vi "Мажор.vi"() -> ()   [LabVIEW 2013]
panel:
  out "output array":dbl[](array[numeric])
  out "s? t:f":dbl
  out "element":dbl
  out "После ошибки":dbl[](array[numeric])
  out "2-х массив на выходе 3":dbl[][](array[numeric])
  out "x*y":i32
  out "size(s)":i32
  in  "Размер окна":i32=4
  out "см. 1.5":dbl[][](array[numeric])
  out "Декодированное сообщение":dbl[](array[numeric])
  out "Детектированное сообщение":dbl[](array[numeric])
  out "Numeric":dbl
  out "Numeric 2":dbl
  out "До ошибки":dbl[](array[numeric])
  in  "Кол-во копий":i32=5
  out "Массиве":dbl[](array[numeric])
  in  "Кол-во элементов":i32=16
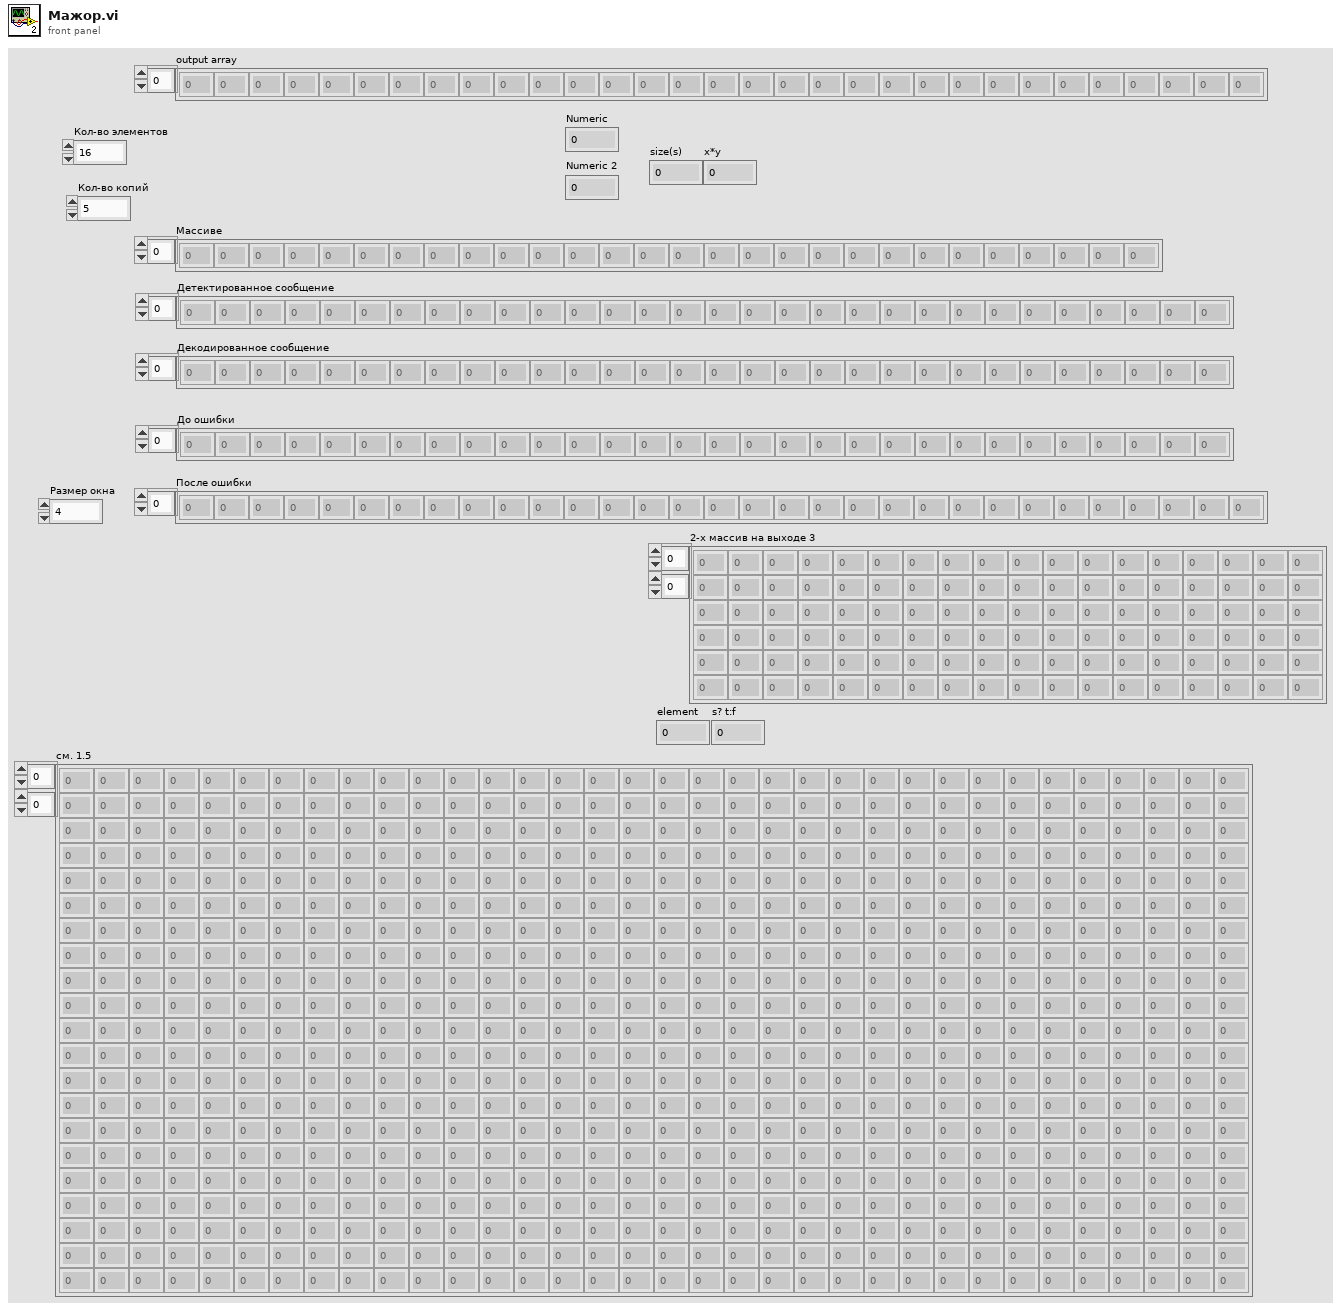
[diagram p1: front panel]
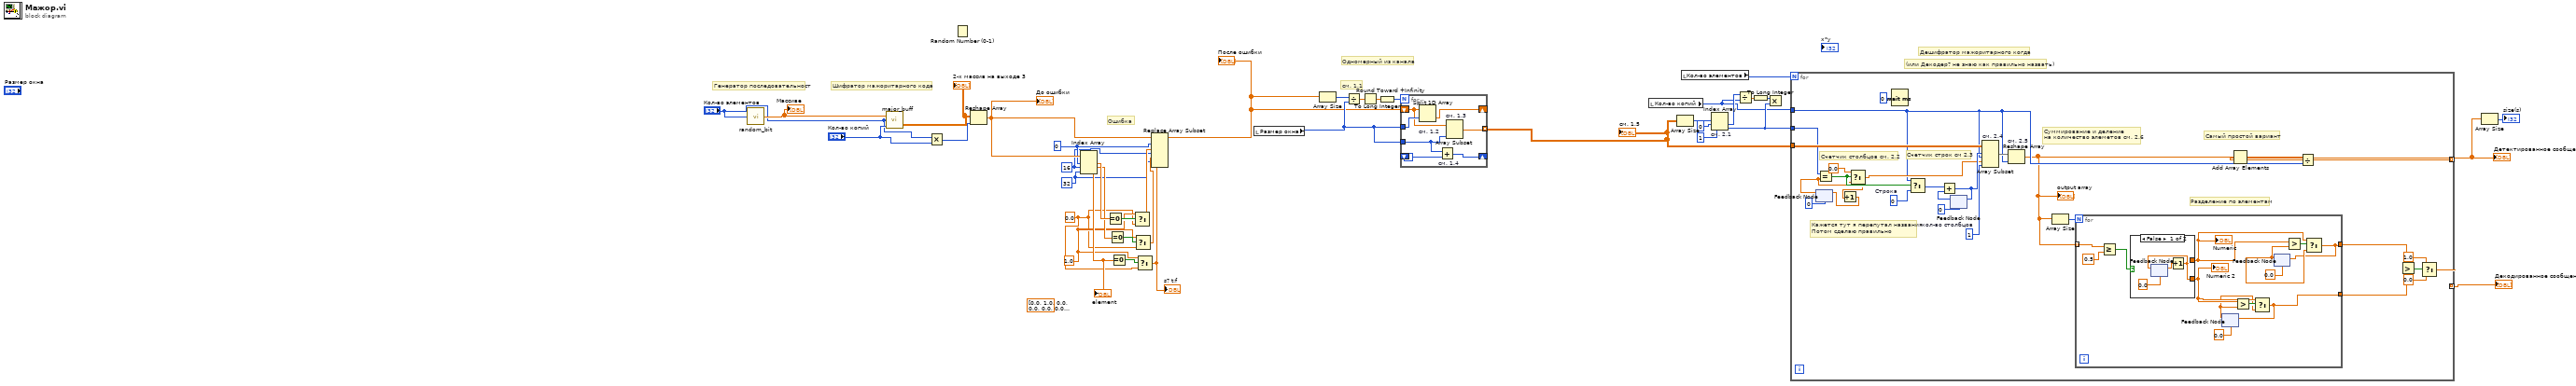
[diagram p0: block diagram]
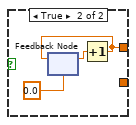
[diagram p2: hidden frame]
diagram:
  (unwired) dbl[] [0.0, 1.0, 0.0, 0.0, 0.0, 0.0, 0.0, 1.0, 1.0, 1.0, 0.0, 1.0, 1.0, 0.0, 0.0, 1.0] ("Декодированное сообщение")
  w8 = 1.0
  w7 = 0.0
  w1 = 32
  w2 = 16
  w3 = 0
  # "Ошибка"
  # "Одномерный из канала"
  # "см. 1.1"
  # "(или Декодер? не знаю как правильно назвать)"
  # "Дешифратор мажоритарного когда"
  # "Шифратор мажоритарного кода"
  # "Генератор последовательност"
  n1 = call "random_bit.vi"("Количество бит"="Кол-во элементов") -> ("Биты на выходе 1"=w39:dbl[])
  "Массиве" <- w39
  n2 = call "major_buff.vi"("Кол-во копий"="Кол-во копий", "Размер окна"="Кол-во элементов", "Биты на выходе 1"=w39) -> ("Подготовленный к отправке мажоритарный код"=w17:dbl[][])  [unwired: 1 out]
  "2-х массив на выходе 3" <- w17
  n3 = Multiply(x="Кол-во элементов", y="Кол-во копий") -> (x*y=w38:i32)
  n4 = Random Number (0-1)() -> ()  [unwired: 1 out]
  n5 = Reshape Array(w17, w38) -> (w15:dbl[])
  "До ошибки" <- w15
  n6 = Index Array(array=w15, index #1=w3, index #2=w2, index #3=w1) -> (element #1=w14:dbl, element #2=w13:dbl, element #3=w12:dbl)
  "element" <- w12
  n7 = Equal To 0?(x=w14) -> (x = 0?=w11:bool)
  n8 = Equal To 0?(x=w13) -> (x = 0?=w10:bool)
  n9 = Equal To 0?(x=w12) -> (x = 0?=w9:bool)
  n10 = Select(t=w8, s=w11, f=w7) -> (s? t:f=w6:dbl)
  n11 = Select(t=w8, s=w10, f=w7) -> (s? t:f=w5:dbl)
  n12 = Select(t=w8, s=w9, f=w7) -> (s? t:f=w4:dbl)
  "s? t:f" <- w4
  n13 = Replace Array Subset(array=w15, new element #1=w6, index #1=w3, new element #2=w5, index #2=w2, new element #3=w4, index #3=w1) -> (w20:dbl[])
  "После ошибки" <- w20
  n14 = local read "Размер окна"() -> (w28:i32)
  n15 = Array Size(array=w20) -> (size(s)=w27:i32)
  n16 = Divide(x=w27, y=w28) -> (x/y=w26:dbl)
  n17 = Round Toward +Infinity(x=w26) -> (ceil(x): smallest int >= x=w25:dbl)
  n18 = To Long Integer(number=w25) -> (32bit integer=w24:i32)
  n19 = for {
    N: w24 -> [_]
    shift-right: [w46] -> _
    shift-left: w20 -> [w44]
    tunnel: w28 -> [w45]
    shift-right: [w42] -> _
    shift-left: _ -> [w41]
    tunnel: w28 -> [w43]
    tunnel: [w40] -> w16 mode=indexing
    n20 = Split 1D Array "см. 1.2"(array=w44, index=w45) -> (second subarray=w46:dbl[])  [unwired: 1 out]
    n21 = Add "см. 1.4"(x=w43, y=w41) -> (x+y=w42:i32)
    n22 = Array Subset "см. 1.3"(array=w44, length=w43) -> (w40:dbl[])  [unwired: 1 in]
  }
  "см. 1.5" <- w16
  n23 = local read "Кол-во копий"() -> (w30:i32)
  n24 = Array Size(array=w16) -> (size(s)=w37:i32[])
  n25 = local read "Кол-во элементов"() -> (w21:i32)
  n26 = Index Array "см. 2.1"(array=w37, index #1=0 ("index"), index #2=1 ("index")) -> (element #1=w34:i32, element #2=w33:i32)
  n27 = Divide(x=w34, y=w30) -> (x/y=w32:dbl)
  n28 = To Long Integer(number=w32) -> (32bit integer=w31:i32)
  n29 = Multiply(x=w31, y=w33) -> ()  [unwired: 1 out]
  n30 = for {
    N: w21 -> [_]
    tunnel: w16 -> [w72]
    tunnel: w33 -> [w64]
    tunnel: w30 -> [w56]
    tunnel: [w55] -> w23 mode=indexing
    tunnel: [w49] -> w29 mode=indexing
    w71 = 1  # кол-во столбцов
    w62 = 0  # Строка
    # "Разделение по элементам"
    # "Самый простой вариант"
    # "Суммирование и деление \nна количество элеметов см. 2.6"
    # "Кажется тут я перепутал названия  \nПотом сделаю правильно"
    # "Счетчик строк см 2.3"
    # "Счетчик столбцов см. 2.2"
    n31 = feedback #1(0) -> (w60:dbl)
    n32 = Equal?(x=w64, y=w60) -> (x = y?=w66:bool)
    n33 = Select(t=0.0, s=w66, f=w60) -> (s? t:f=w59:dbl)
    n34 = Increment(x=w59) -> (x+1=w58:dbl)
    n35 = feedback-in #1(w58) -> ()
    n36 = Wait (ms)(milliseconds to wait=u32 0) -> ()  [unwired: 1 out]
    n37 = Select(t=w56, s=w66, f=w62) -> (s? t:f=w63:i32)
    n38 = feedback #2(0) -> (w65:i32)
    n39 = Add(x=w63, y=w65) -> (x+y=w61:i32)
    n40 = feedback-in #2(w61) -> ()
    n41 = Array Subset "см. 2.4"(array=w72, index (row)=w61, length (row)=w56, index (col)=w59, length (col)=w71) -> (w73:dbl[][])
    n42 = Reshape Array "см. 2.5"(w73, w56) -> (w53:dbl[])
    "output array" <- w53
    n43 = Array Size(array=w53) -> (size(s)=w54:i32)
    n44 = for {
      N: w54 -> [_]
      tunnel: w53 -> [w84] mode=indexing
      tunnel: [w79] -> w48
      tunnel: [w75] -> w47
      n45 = Greater Or Equal?(x=w84, y=0.5) -> (x >= y?=w85:bool)
      n46 = case shown="False" w85 {
        tunnel: [_ w90] -> w83
        tunnel: [w87 _] -> w82
        frame False {
          n47 = feedback #3(0.0) -> (w88:dbl)
          n48 = Increment(x=w88) -> (x+1=w87:dbl)
          n49 = feedback-in #3(w87) -> ()
        }
        frame True {
          n50 = feedback #4(0.0) -> (w91:dbl)
          n51 = Increment(x=w91) -> (x+1=w90:dbl)
          n52 = feedback-in #4(w90) -> ()
        }
      }
      "Numeric" <- w83
      "Numeric 2" <- w82
      n53 = feedback #5(0.0) -> (w74:dbl)
      n54 = Greater?(x=w82, y=w74) -> (0:w81:bool)
      n55 = Select(t=w82, s=w81, f=w74) -> (s? t:f=w79:dbl)
      n56 = feedback-in #5(w79) -> ()
      n57 = feedback #6(0.0) -> (w77:dbl)
      n58 = Greater?(x=w83, y=w77) -> (0:w78:bool)
      n59 = Select(t=w83, s=w78, f=w77) -> (s? t:f=w75:dbl)
      n60 = feedback-in #6(w75) -> ()
    }
    n61 = Add Array Elements(numeric array=w53) -> (sum=w57:dbl)
    n62 = Divide(x=w57, y=w56) -> (x/y=w55:dbl)
    n63 = Greater?(x=w47, y=w48) -> (0:w52:bool)
    n64 = Select(t=1.0, s=w52, f=0.0) -> (s? t:f=w49:dbl)
  }
  "Детектированное сообщение" <- w23
  "Декодированное сообщение" <- w29
  n65 = Array Size(array=w23) -> (size(s)=→"size(s)":i32)
